vi "Extend Symbol Path.vi"(3 "Symbol Path":path) -> (1 "Resolved Path":path)   [LabVIEW 2017]
doc: "Expands a LabVIEW symbolic path into a real path. Recognised forms include <application>, <desktop>, <temp>, <user.lib>, <vi.lib>, [xxx] custom symbols and %SystemVariable% environment variables."
uses:
  <vilib>/Utility/sysdir.llb/System Directory Type.ctl
panel:
  # "#Note [xxx] or <xxx>\n- [application]\n- [desktop]\n- [temp][temporary]\n- [user.lib]\n- [vi.lib]\n-%SystemVariable%, eg: OneDrive"
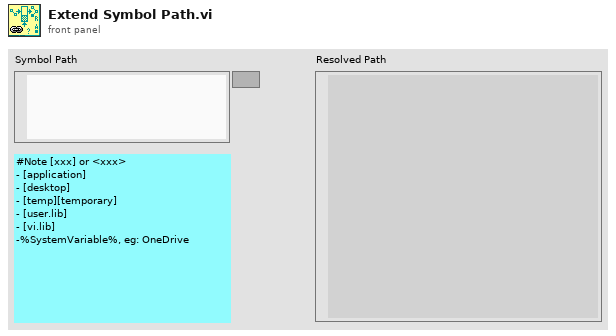
[diagram p1: front panel]
types:
  T1 = enum16{"Absolute path", "Relative path", "<Not A Path>"}
  T2 = typedef "System Directory Type.ctl" = i32
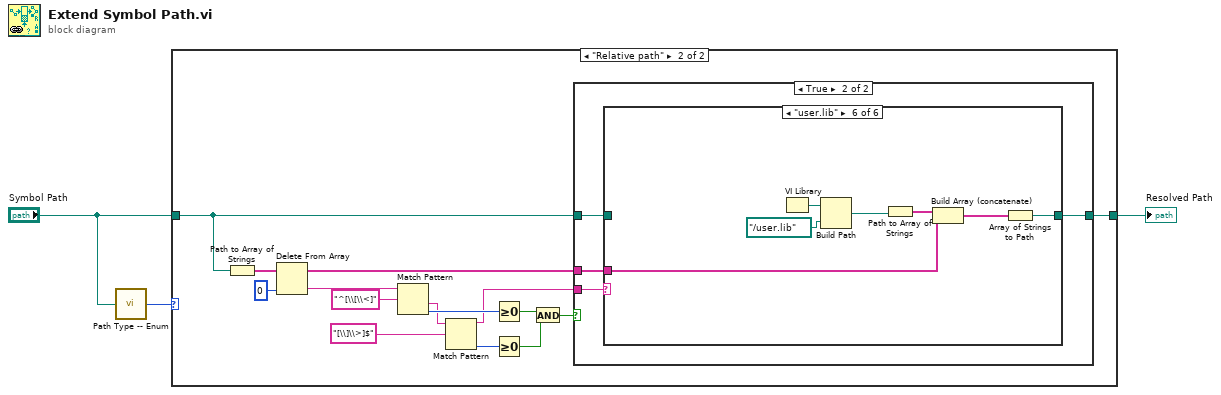
[diagram p0: block diagram]
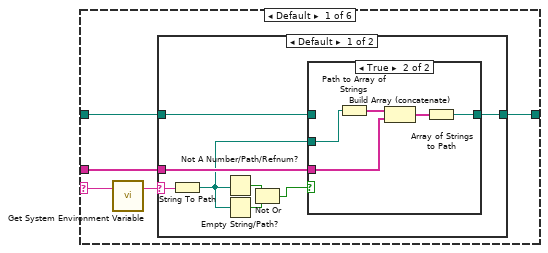
[diagram p4: hidden frame]
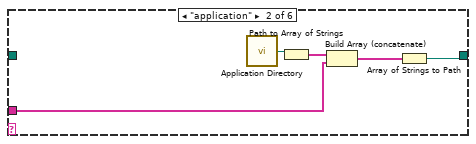
[diagram p7: hidden frame]
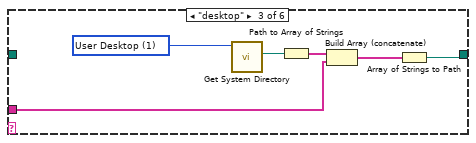
[diagram p8: hidden frame]
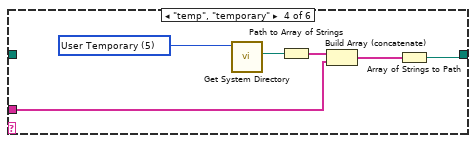
[diagram p9: hidden frame]
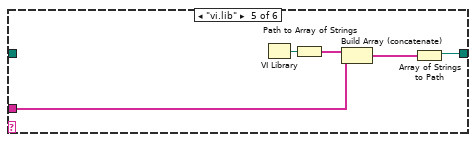
[diagram p10: hidden frame]
diagram:
  n1 = call "Path Type -- Enum.vi"("Value"="Symbol Path") -> ("Enum"=w3:T1)
  n2 = case shown="\"Relative path\"" w3 {
    tunnel: [w4 w11] -> w2
    tunnel: "Symbol Path" -> [w4 w10]
    frame "Absolute path", "<Not A Path>", Default {
    }
    frame "Relative path" {
      n3 = Path to Array of Strings(0:w10) -> (2:w19:string[])  [unwired: 1 out]
      n4 = Delete From Array(array=w19, index=0) -> (deleted portion=w9:string, array with subset deleted=w5:string[])  [unwired: 1 in]
      n5 = Match Pattern(string=w9, regular expression="^[\\[\\<]") -> (after substring=w8:string, offset past match=w16:i32)  [unwired: 1 in, 2 out]
      n6 = Match Pattern(string=w8, regular expression="[\\]\\>]$") -> (before substring=w7:string, offset past match=w15:i32)  [unwired: 1 in, 2 out]
      n7 = Greater Or Equal To 0?(x=w16) -> (x >= 0?=w14:bool)
      n8 = Greater Or Equal To 0?(x=w15) -> (x >= 0?=w13:bool)
      n9 = And(x=w14, y=w13) -> (x .and. y?=w12:bool)
      n10 = case shown="True" w12 {
        tunnel: [w20 w21] -> w11
        tunnel: w10 -> [w20 w23]
        tunnel: w7 -> [_ w24]
        tunnel: w5 -> [_ w22]
        frame False {
        }
        frame True {
          n11 = case shown="\"user.lib\"" w24 {
            selector: w24 -> [w29 _ _ _ _ _]
            tunnel: w23 -> [w26 _ _ _ _ _]
            tunnel: w22 -> [w25 w45 w52 w58 w62 w69]
            tunnel: [w27 w47 w53 w59 w64 w71] -> w21
            frame Default {
              n12 = call "Get System Environment Variable.vi"("Environment Variable Name"=w29) -> ("Value"=w28:string)  [unwired: 2 in]
              n13 = case shown="Default" w28 {
                selector: w28 -> [w37 _]
                tunnel: [w35 w44] -> w27
                tunnel: w26 -> [w34 w44]
                tunnel: w25 -> [w33 _]
                frame Default {
                  n14 = String To Path(string=w37) -> (path=w32:path)
                  n15 = Not A Number/Path/Refnum?(number/path/refnum=w32) -> (NaN/Path/Refnum?=w31:bool)
                  n16 = Empty String/Path?(string/path=w32) -> (empty?=w30:bool)
                  n17 = Not Or(1:w30, 2:w31) -> (0:w36:bool)
                  n18 = case shown="True" w36 {
                    tunnel: [w38 w41] -> w35
                    tunnel: w34 -> [w38 _]
                    tunnel: w33 -> [_ w40]
                    tunnel: w32 -> [_ w39]
                    frame False {
                    }
                    frame True {
                      n19 = Path to Array of Strings(0:w39) -> (2:w42:string[])  [unwired: 1 out]
                      n20 = Build Array (concatenate)(w42, w40) -> (w43:string[])
                      n21 = Array of Strings to Path(0:w43) -> (2:w41:path)  [unwired: 1 in]
                    }
                  }
                }
                frame "" {
                }
              }
            }
            frame "application" {
              n22 = call <vilib>:"Application Directory.vi"() -> ("Application Directory"=w46:path)
              n23 = Path to Array of Strings(0:w46) -> (2:w48:string[])  [unwired: 1 out]
              n24 = Build Array (concatenate)(w48, w45) -> (w49:string[])
              n25 = Array of Strings to Path(0:w49) -> (2:w47:path)  [unwired: 1 in]
            }
            frame "desktop" {
              w51 = T2 1 items=["User Home"=0, "User Desktop"=1, "User Documents"=2, "User Application Data"=3, "User Preferences"=4, "User Temporary"=5, "Public Documents"=6, "Public Application Data"=7, "Public Preferences"=8, "Public Cache"=13, "System Core Libraries"=9, "System Installed Libraries"=10, "Application Files"=11, "Boot Volume Root"=12] ("system directory type")
              n26 = call <vilib>:"Get System Directory.vi"("system directory type"=w51) -> ("system directory"=w50:path)  [unwired: 10 in]
              n27 = Path to Array of Strings(0:w50) -> (2:w54:string[])  [unwired: 1 out]
              n28 = Build Array (concatenate)(w54, w52) -> (w55:string[])
              n29 = Array of Strings to Path(0:w55) -> (2:w53:path)  [unwired: 1 in]
            }
            frame "temp", "temporary" {
              w57 = T2 5 items=["User Home"=0, "User Desktop"=1, "User Documents"=2, "User Application Data"=3, "User Preferences"=4, "User Temporary"=5, "Public Documents"=6, "Public Application Data"=7, "Public Preferences"=8, "Public Cache"=13, "System Core Libraries"=9, "System Installed Libraries"=10, "Application Files"=11, "Boot Volume Root"=12] ("system directory type")
              n30 = call <vilib>:"Get System Directory.vi"("system directory type"=w57) -> ("system directory"=w56:path)  [unwired: 10 in]
              n31 = Path to Array of Strings(0:w56) -> (2:w60:string[])  [unwired: 1 out]
              n32 = Build Array (concatenate)(w60, w58) -> (w61:string[])
              n33 = Array of Strings to Path(0:w61) -> (2:w59:path)  [unwired: 1 in]
            }
            frame "vi.lib" {
              n34 = VI Library() -> (path=w63:path)
              n35 = Path to Array of Strings(0:w63) -> (2:w65:string[])  [unwired: 1 out]
              n36 = Build Array (concatenate)(w65, w62) -> (w66:string[])
              n37 = Array of Strings to Path(0:w66) -> (2:w64:path)  [unwired: 1 in]
            }
            frame "user.lib" {
              n38 = VI Library() -> (path=w68:path)
              n39 = Build Path(base path=w68, name or relative path=path "../user.lib" ("Relative path (.)")) -> (appended path=w70:path)
              n40 = Path to Array of Strings(0:w70) -> (2:w72:string[])  [unwired: 1 out]
              n41 = Build Array (concatenate)(w72, w69) -> (w73:string[])
              n42 = Array of Strings to Path(0:w73) -> (2:w71:path)  [unwired: 1 in]
            }
          }
        }
      }
    }
  }
  "Resolved Path" <- w2
